vi "System Exec Output to String Indicator.vi"() -> ()   [LabVIEW 2011]
panel:
  out "standard output":string
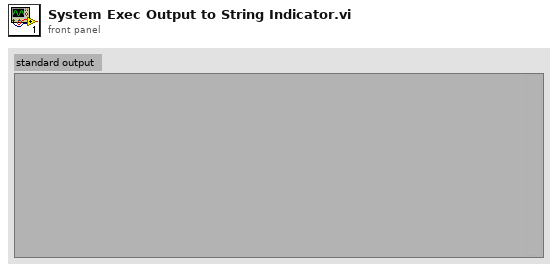
[diagram p1: front panel]
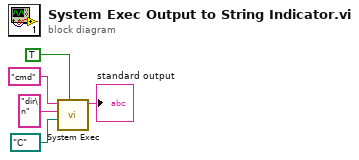
[diagram p0: block diagram]
diagram:
  n1 = call <vilib>:"System Exec.vi"("wait until completion? (T)"=TRUE, "working directory"=path "C:/", "standard input"="dir\n", "command line"="cmd") -> ("standard output"=→"standard output":string)  [unwired: 4 in, 3 out]
